vi "Agilent SNA Set Power Sweep.vi"(7 "Agilent SNA & SWP":T1, 8 "error in (no error)":errorcluster, 10 "Start/Stop Power, dBm":cluster{"Pstart":dbl, "Pstop":dbl}, 11 "VISA Resource Names":T2) -> (0 "error out":errorcluster, 3 "dup VISA Resource Names":T2)   [LabVIEW 2011]
doc: "This vi sets the power range. Only works on the HP 8753D."
uses:
  TypeDefs/Agilent SNA VISA.ctl
  TypeDefs/Agilent SNA Instrument Info.ctl
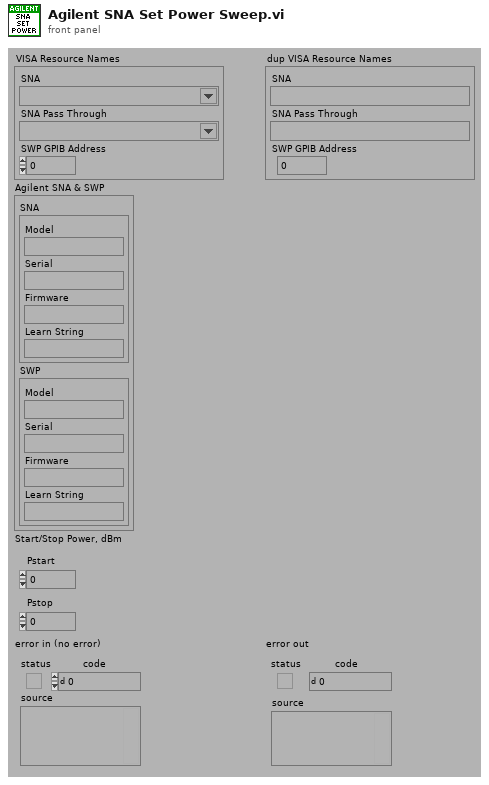
[diagram p1: front panel]
types:
  T1 = typedef "Agilent SNA Instrument Info.ctl" = cluster{"SNA":cluster{"Model":string, "Serial":string, "Firmware":string, "Learn String":string}, "SWP":cluster{"Model":string, "Serial":string, "Firmware":string, "Learn String":string}}
  T2 = typedef "Agilent SNA VISA.ctl" = cluster{"SNA":refnum<visa-resource-name>, "SNA Pass Through":refnum<visa-resource-name>, "SWP GPIB Address":i32}
  T3 = typedef "Agilent SNA Model.ctl" = enum16{"Not Supported", "8757X"}
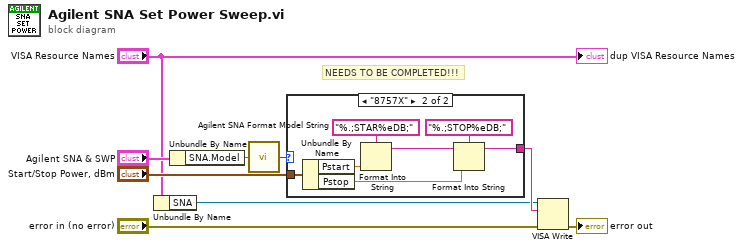
[diagram p0: block diagram]
diagram:
  # "NEEDS TO BE COMPLETED!!!"
  n1 = Unbundle By Name("VISA Resource Names") -> ("SNA"=w1:refnum<visa-resource-name>)
  n2 = Unbundle By Name("Agilent SNA & SWP") -> ("SNA.Model"=w4:string)
  n3 = call "Agilent SNA Format Model String.vi"("Model String"=w4) -> ("Model"=w3:T3)
  n4 = case shown="\"8757X\"" w3 {
    tunnel: "Start/Stop Power, dBm" -> [_ w15]
    tunnel: [_ w10] -> w6
    frame "Not Supported" {
    }
    frame "8757X" {
      n5 = Unbundle By Name(w15) -> ("Pstart"=w12:dbl, "Pstop"=w11:dbl)
      n6 = Format Into String(format string="%.;STAR%eDB;", w12) -> (resulting string=w13:string)  [unwired: 2 in, 1 out]
      n7 = Format Into String(format string="%.;STOP%eDB;", initial string=w13, w11) -> (resulting string=w10:string)  [unwired: 1 in, 1 out]
    }
  }
  n8 = VISA Write(VISA resource name=w1, write buffer=w6, error in (no error)="error in (no error)") -> (error out=→"error out":errorcluster)  [unwired: 2 out]
  "dup VISA Resource Names" <- "VISA Resource Names"
